vi "GetResponse.vi"(3 "error in":errorcluster, 4 "Delay Time (s)":dbl, 5 "Validate Checksum":bool) -> (0 "error out":errorcluster, 1 "Status":bool, 2 "Receive_buffer out":u8[](array[numeric]))   [LabVIEW 2014]
panel:
  out "Read Time":u32
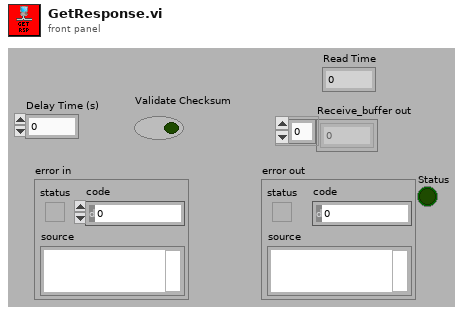
[diagram p1: front panel]
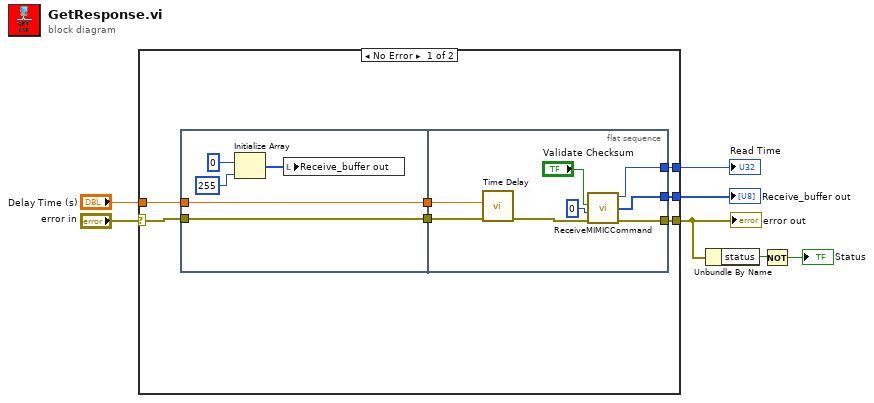
[diagram p0: block diagram]
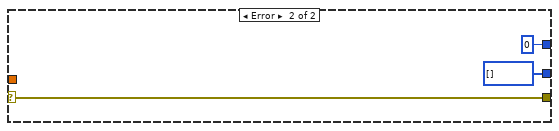
[diagram p2: hidden frame]
diagram:
  n1 = case shown="No Error" "error in" {
    selector: "error in" -> [w14 w30]
    tunnel: [w12 w30] -> w4
    tunnel: "Delay Time (s)" -> [w13 _]
    tunnel: [w9 u8[] [] ("Receive_buffer")] -> w5
    tunnel: [w8 u32 0 ("Read Time")] -> w3
    frame No Error {
      n2 = flat-sequence {
        tunnel: w13 -> [w18]
        tunnel: w14 -> [w19]
        tunnel: [w19] -> w11
        tunnel: [w18] -> w10
        tunnel: [w24] -> w12
        tunnel: w11 -> [w27]
        tunnel: w10 -> [w26]
        tunnel: [w23] -> w9
        tunnel: [w22] -> w8
        frame #0 {
          n3 = Initialize Array(u8 0 ("element"), 255 ("dimension size")) -> (w17:u8[])
          n4 = local write "Receive_buffer out"(w17) -> ()
        }
        frame #1 {
          n5 = call "Time Delay"("error in (no error)"=w27, "Delay Time (s)"=w26) -> ("error out"=w25:errorcluster)  [unwired: 9 in]
          n6 = call "ReceiveMIMICCommand.vi"("error in"=w25, "Desired_Length"=u32 0, "CheckSum?"="Validate Checksum") -> ("Receive_buffer"=w23:u8[], "error out"=w24:errorcluster, "Read Time"=w22:u32)  [unwired: 1 in, 2 out]
        }
      }
    }
    frame Error {
    }
  }
  "error out" <- w4
  "Receive_buffer out" <- w5
  "Read Time" <- w3
  n7 = Unbundle By Name(w4) -> ("status"=w2:bool)
  n8 = Not(x=w2) -> (.not. x?=→"Status":bool)
